vi "GetRemoteTasklist.vi"(8 "error in (no error)":errorcluster, 11 "Input IP Address":string) -> (0 "error out":errorcluster, 1 "standard error":string, 3 "Open Devices":string[](array[string]))   [LabVIEW 2020]
uses:
  <vilib>/regexp/Match Regular Expression.xnode
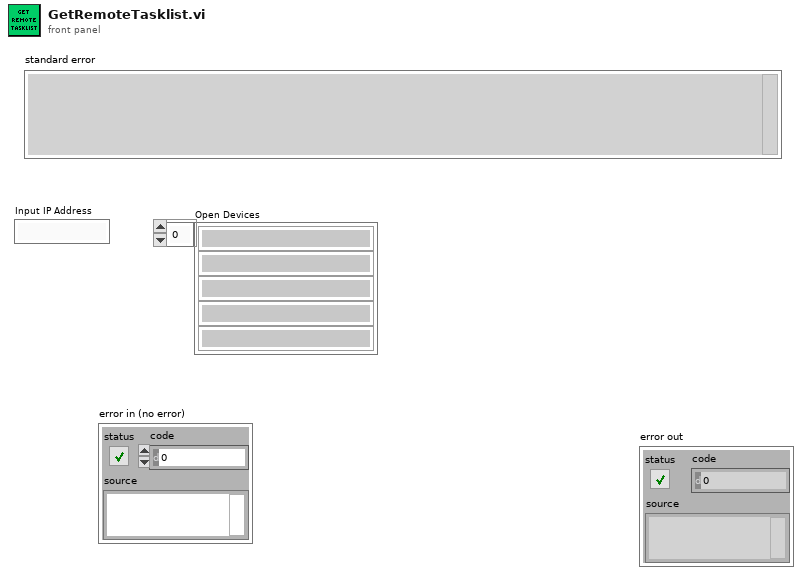
[diagram p1: front panel]
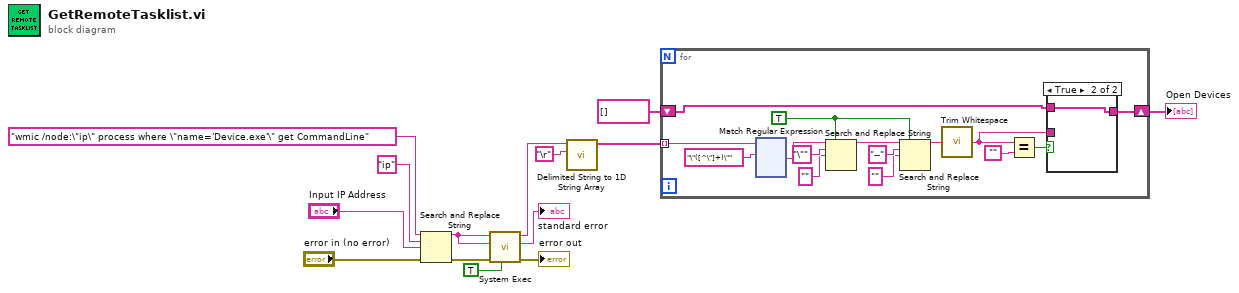
[diagram p0: block diagram]
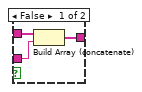
[diagram p2: hidden frame]
diagram:
  n1 = Search and Replace String(input string="wmic /node:\"ip\" process where \"name='Device.exe'\" get CommandLine" ("command line"), search string="ip", replace string="Input IP Address", error in="error in (no error)") -> (result string=w10:string, error out=w2:errorcluster)  [unwired: 4 in, 2 out]
  n2 = call <vilib>:"System Exec.vi"("run minimized? (F)"=TRUE, "error in (no error)"=w2, "standard input"=w10, "command line"=w10) -> ("error out"=→"error out":errorcluster, "standard error"=→"standard error":string, "standard output"=w7:string)  [unwired: 4 in, 1 out]
  n3 = call <vilib>:"Delimited String to 1D String Array.vi"("delimiter"="\r", "delimited string"=w7) -> ("string array"=w8:string[])  [unwired: 9 in]
  n4 = for {
    tunnel: w8 -> [w28] mode=indexing
    shift-right: [w18] -> w5
    shift-left: string[] [] -> [w15]
    w21 = TRUE ("replace all? (F)")
    n5 = xnode "Match Regular Expression"("input string"=w28, "regular expression"="\"([^\"]+)\"") -> ("after match"=w22:string)  [unwired: 4 in, 4 out]
    n6 = Search and Replace String(replace all?=w21, input string=w22, search string="\"", replace string="" ("replace string (\"\")")) -> (result string=w25:string)  [unwired: 4 in, 3 out]
    n7 = Search and Replace String(replace all?=w21, input string=w25, search string="--", replace string="" ("replace string (\"\")")) -> (result string=w20:string)  [unwired: 4 in, 3 out]
    n8 = call <vilib>:"Trim Whitespace.vi"("string"=w20) -> ("trimmed string"=w17:string)  [unwired: 1 in]
    n9 = Equal?(x=w17, y="") -> (x = y?=w16:bool)
    n10 = case shown="True" w16 {
      tunnel: [w32 w33] -> w18
      tunnel: w17 -> [w30 _]
      tunnel: w15 -> [w31 w33]
      frame False {
        n11 = Build Array (concatenate)(w31, w30) -> (w32:string[])
      }
      frame True {
      }
    }
  }
  "Open Devices" <- w5
